vi "Saturation Compensator.vi"(7 "Saturation Commands":dbl[](array[numeric]), 10 "Voltage Commands":dbl[](array[numeric])) -> (3 "Saturated Voltage":dbl[](array[numeric]))   [LabVIEW 2017]
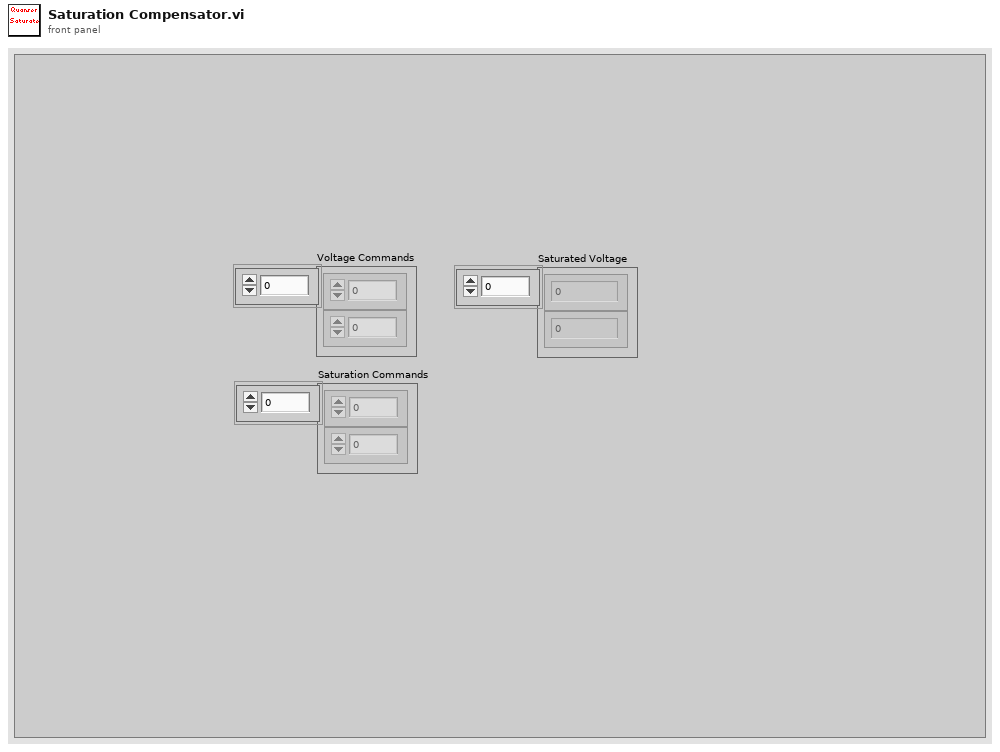
[diagram p1: front panel]
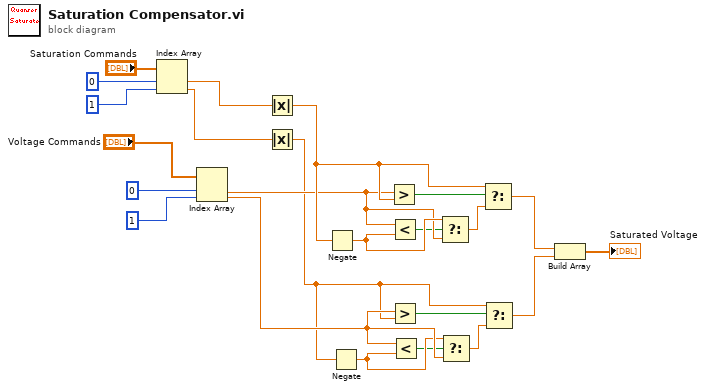
[diagram p0: block diagram]
diagram:
  n1 = Index Array(array="Saturation Commands", index #1=0 ("index"), index #2=1 ("index 2")) -> (element #1=w3:dbl, element #2=w2:dbl)
  n2 = Index Array(array="Voltage Commands", index #1=0 ("index"), index #2=1 ("index 2")) -> (element #1=w13:dbl, element #2=w22:dbl)
  n3 = Absolute Value(x=w3) -> (abs(x)=w20:dbl)
  n4 = Absolute Value(x=w2) -> (abs(x)=w1:dbl)
  n5 = Negate(x=w20) -> (-x=w15:dbl)
  n6 = Negate(x=w1) -> (-x=w21:dbl)
  n7 = Greater?(x=w13, y=w20) -> (0:w8:bool)
  n8 = Less?(x=w13, y=w15) -> (x < y?=w12:bool)
  n9 = Greater?(x=w22, y=w1) -> (0:w16:bool)
  n10 = Less?(x=w22, y=w21) -> (x < y?=w17:bool)
  n11 = Select(t=w15, s=w12, f=w13) -> (s? t:f=w14:dbl)
  n12 = Select(t=w21, s=w17, f=w22) -> (s? t:f=w18:dbl)
  n13 = Select(t=w20, s=w8, f=w14) -> (s? t:f=w7:dbl)
  n14 = Select(t=w1, s=w16, f=w18) -> (s? t:f=w19:dbl)
  n15 = Build Array(w7, w19) -> (→"Saturated Voltage":dbl[])
